vi "Sel_files_filter.vi"(8 "error in":errorcluster, 10 "Filter":string[](array[string]), 11 "path":path) -> (3 "String Array Matched":string[](array[string])=["c:\\DATA\\20141011-102717-0.fits", "c:\\DATA\\20141011-102717-1.fits"], 5 "number of found":i32)   [LabVIEW 2012]
panel:
  out "number of dirs found":i32
  out "String Array Matched":string[](array[string])=["c:\\DATA\\20141011-102717-0.fits", "c:\\DATA\\20141011-102717-1.fits"]
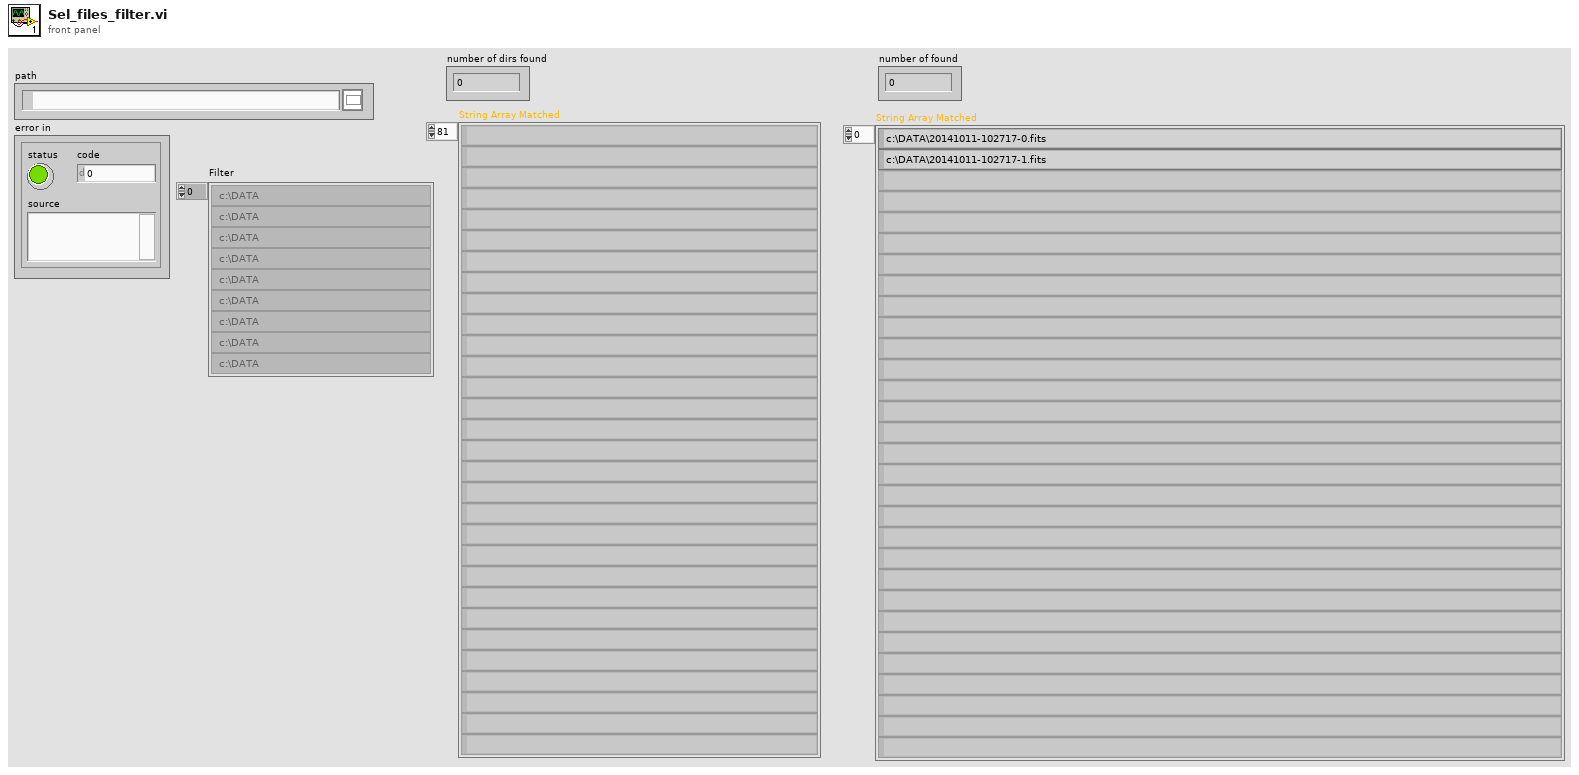
[diagram p1: front panel]
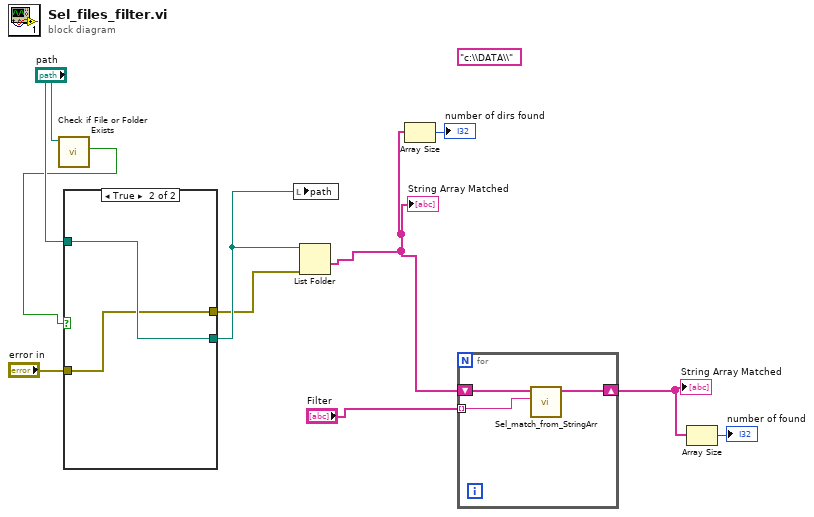
[diagram p0: block diagram]
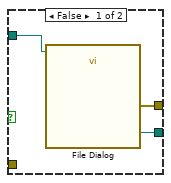
[diagram p2: hidden frame]
diagram:
  (unwired) "c:\\DATA\\"
  n1 = call <vilib>:"Check if File or Folder Exists.vi"("path"="path") -> ("file or folder exists?"=w4:bool)  [unwired: 8 in, 2 out]
  n2 = case shown="True" w4 {
    tunnel: [w13 w15] -> w10
    tunnel: "path" -> [w12 w15]
    tunnel: [w11 w14] -> w3
    tunnel: "error in" -> [_ w14]
    frame False {
      n3 = call "File Dialog"("start path"=w12) -> ("selected path"=w13:path, "error out"=w11:errorcluster)  [unwired: 11 in, 2 out]
    }
    frame True {
    }
  }
  n4 = local write "path"(w10) -> ()
  n5 = List Folder(path=w10, error in=w3) -> (folder names=w7:string[])  [unwired: 2 in, 3 out]
  "String Array Matched" <- w7
  n6 = Array Size(array=w7) -> (size(s)=→"number of dirs found":i32)
  n7 = for {
    shift-right: [w18] -> w9
    shift-left: w7 -> [w17]
    tunnel: "Filter" -> [w16] mode=indexing
    n8 = call "Sel_match_from_StringArr.vi"("String to match"=w16, "String Array In"=w17) -> ("String Array Matched"=w18:string[])  [unwired: 7 in, 2 out]
  }
  "String Array Matched" <- w9
  n9 = Array Size(array=w9) -> (size(s)=→"number of found":i32)
